vi "Output Configuration (Read).vi"(6 "ISOBUS address":T3=-1 caption="ISOBUS address (-1)", 8 "error in":errorcluster, 11 "Mercury Reference In":T4) -> (0 "error out":errorcluster, 2 "Out Config":T1="SERS" caption="Output Configuration", 3 "Mercury Reference Out":T4, 4 "Valid?":T2)   [LabVIEW 2014, in "Mercury iXX.lvlib" / "Magnet.lvlib"]
doc: "Read the output configuration of the magnet PSU."
uses:
  Magnet.lvlib
  Controls/Mercury Reference.ctl
  Controls/Comms Transport Layer.ctl
  Private/Controls/Query Dynamic Reference.ctl
  Controls/ISOBus Address.ctl
  Controls/Is Valid LED.ctl
  Controls/Output Configuration.ctl
  Private/Controls/Command Verbs.ctl
  Mercury iXX.lvlib
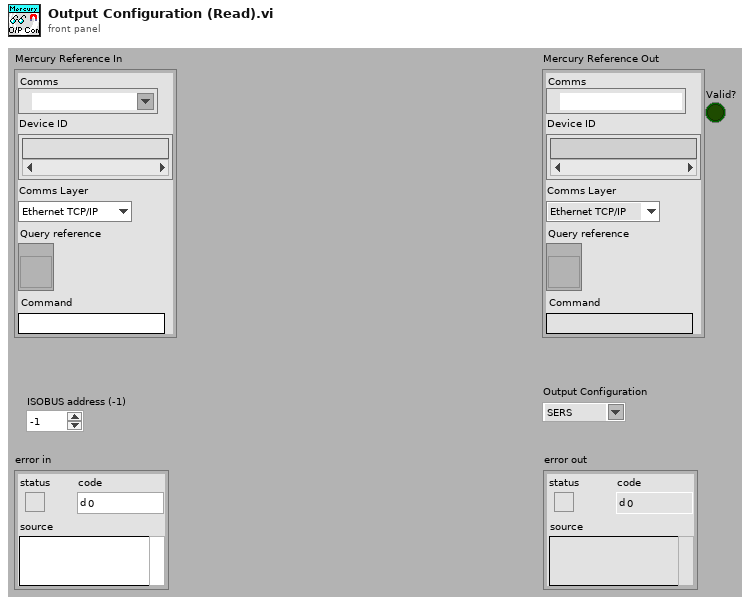
[diagram p1: front panel]
types:
  T1 = typedef "Mercury iXX.lvlib/Magnet.lvlib/Output Configuration.ctl" = string
  T2 = typedef "Mercury iXX.lvlib/Is Valid LED.ctl" = bool
  T3 = typedef "Mercury iXX.lvlib/ISOBus Address.ctl" = i32
  T4 = typedef "Mercury iXX.lvlib/Mercury Reference.ctl" = cluster{"Comms":refnum<visa-resource-name>, "Device ID":string[], "Comms Layer":T5, "Command":string, "Query reference":T6}
  T5 = typedef "Mercury iXX.lvlib/Comms Transport Layer.ctl" = enum16{"Ethernet TCP/IP", "USB", "ISOBus - RS-232", "GPIB"}
  T6 = typedef "Mercury iXX.lvlib/Query Dynamic Reference.ctl" = refnum<vi>
  T7 = typedef "Mercury iXX.lvlib/Command Verbs.ctl" = string
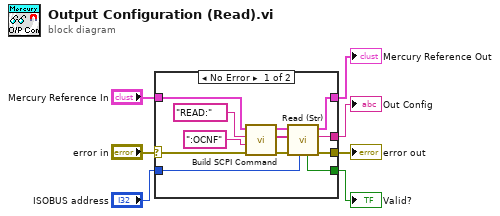
[diagram p0: block diagram]
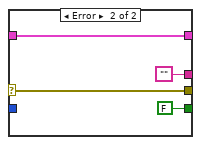
[diagram p2: hidden frame]
diagram:
  n1 = case shown="No Error" "error in" {
    selector: "error in" -> [w18 w22]
    tunnel: "Mercury Reference In" -> [w19 w23]
    tunnel: "ISOBUS address" -> [w14 _]
    tunnel: [w13 T2 FALSE ("Valid?")] -> w5
    tunnel: [w12 w22] -> w4
    tunnel: [w10 w23] -> w3
    tunnel: [w11 ""] -> w2
    frame No Error {
      n2 = call "Build SCPI Command.vi"("error in"=w18, "Noun(s)"=":OCNF" ("Command"), "Verb"=T7 "READ:", "Mercury Reference In"=w19) -> ("error out"=w8:errorcluster, "SCPI Message(s)"=w9:string[], "Mercury Reference Out"=w15:T4)  [unwired: 5 out]
      n3 = call "Read (Str).vi"("ISOBUS address"=w14, "error in"=w8, "SCPI Message(s)"=w9, "Mercury Reference In"=w15) -> ("error out"=w12:errorcluster, "Response"=w11:string, "Mercury Reference Out"=w10:T4, "Valid?"=w13:T2)  [unwired: 4 out]
    }
    frame Error {
    }
  }
  "Mercury Reference Out" <- w3
  "error out" <- w4
  "Valid?" <- w5
  "Out Config" <- w2
